vi "Broadcast Refnum Release.vi"(8 "error in":errorcluster) -> (0 "error out":errorcluster)   [LabVIEW 2020, in "SECS Scenarios.lvlib" / "Scenarios Class.lvclass"]
uses:
  Scenarios Class.lvclass
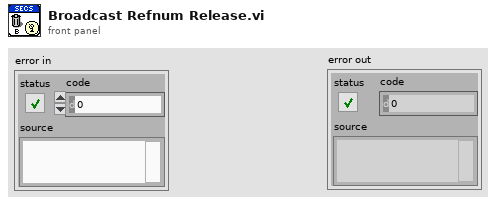
[diagram p1: front panel]
types:
  T1 = typedef "SECS Scenarios.lvlib/Scenarios Class.lvclass/Broadcast Refnum.ctl" = cluster{"13-EnableDisable Alarm":refnum<user-event>, "15-Process Program Request":refnum<user-event>, "16-Process Program Send":refnum<user-event>, "17-Deleting a Process Program by Host":refnum<user-event>, "18-Host Requests Equipment Process Program Directory":refnum<user-event>, "19-Equipment Process Program Uploading":refnum<user-event>, "20[1]-Process Program Downloading":refnum<user-event>, "20[2]-Process Program Downloading":refnum<user-event>, "22-Host Sends Information to Equipment":refnum<user-event>, "26-Host Requests to Enter OFF-Line":refnum<user-event>, "27-Host Requests to Enter On-Line":refnum<user-event>, "28[1]-Remote Control[PP-SELECT]":refnum<user-event>, "28[2]-Remote Control[START]":refnum<user-event>, "28[3]-Remote Control[STOP]":refnum<user-event>, "28[4]-Remote Control[LOCAL]":refnum<user-event>, "28[5]-Remote Control[REMOTE]":refnum<user-event>, "28[6]-Remote Control[RCMD]":refnum<user-event>, "30-Host Requests Equipment to Set Time":refnum<user-event>, "31-Host Requests Time Value from Equipment":refnum<user-event>, "32[1]-Trace Data Collection":refnum<user-event>, "32[2]-Trace Data Collection":refnum<user-event>}
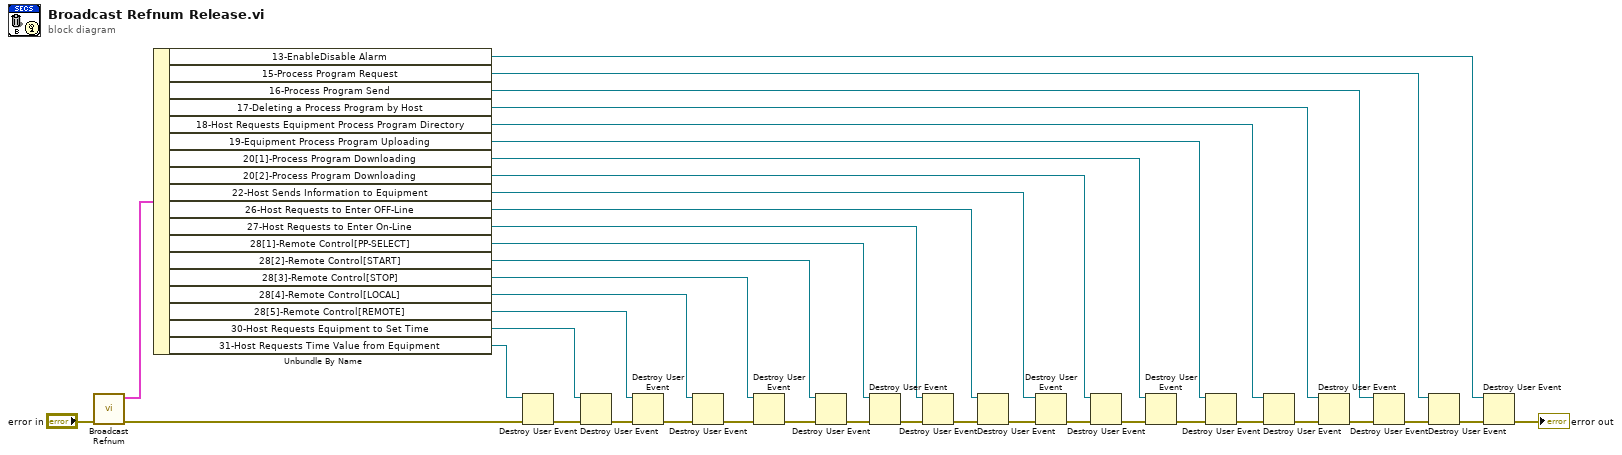
[diagram p0: block diagram]
diagram:
  n1 = call "Broadcast Refnum.vi"("error in"="error in") -> ("error out"=w1:errorcluster, "Broadcast Refnum"=w39:T1)  [unwired: 9 in]
  n2 = Unbundle By Name(w39) -> ("13-EnableDisable Alarm"=w35:refnum<user-event>, "15-Process Program Request"=w37:refnum<user-event>, "16-Process Program Send"=w29:refnum<user-event>, "17-Deleting a Process Program by Host"=w30:refnum<user-event>, "18-Host Requests Equipment Process Program Directory"=w31:refnum<user-event>, "19-Equipment Process Program Uploading"=w21:refnum<user-event>, "20[1]-Process Program Downloading"=w24:refnum<user-event>, "20[2]-Process Program Downloading"=w25:refnum<user-event>, "22-Host Sends Information to Equipment"=w26:refnum<user-event>, "26-Host Requests to Enter OFF-Line"=w18:refnum<user-event>, "27-Host Requests to Enter On-Line"=w16:refnum<user-event>, "28[1]-Remote Control[PP-SELECT]"=w14:refnum<user-event>, "28[2]-Remote Control[START]"=w12:refnum<user-event>, "28[3]-Remote Control[STOP]"=w10:refnum<user-event>, "28[4]-Remote Control[LOCAL]"=w8:refnum<user-event>, "28[5]-Remote Control[REMOTE]"=w6:refnum<user-event>, "30-Host Requests Equipment to Set Time"=w4:refnum<user-event>, "31-Host Requests Time Value from Equipment"=w2:refnum<user-event>)
  n3 = Destroy User Event(user event=w2, error in=w1) -> (error out=w3:errorcluster)
  n4 = Destroy User Event(user event=w4, error in=w3) -> (error out=w5:errorcluster)
  n5 = Destroy User Event(user event=w6, error in=w5) -> (error out=w7:errorcluster)
  n6 = Destroy User Event(user event=w8, error in=w7) -> (error out=w9:errorcluster)
  n7 = Destroy User Event(user event=w10, error in=w9) -> (error out=w11:errorcluster)
  n8 = Destroy User Event(user event=w12, error in=w11) -> (error out=w13:errorcluster)
  n9 = Destroy User Event(user event=w14, error in=w13) -> (error out=w15:errorcluster)
  n10 = Destroy User Event(user event=w16, error in=w15) -> (error out=w17:errorcluster)
  n11 = Destroy User Event(user event=w18, error in=w17) -> (error out=w19:errorcluster)
  n12 = Destroy User Event(user event=w26, error in=w19) -> (error out=w27:errorcluster)
  n13 = Destroy User Event(user event=w25, error in=w27) -> (error out=w28:errorcluster)
  n14 = Destroy User Event(user event=w24, error in=w28) -> (error out=w23:errorcluster)
  n15 = Destroy User Event(user event=w21, error in=w23) -> (error out=w22:errorcluster)
  n16 = Destroy User Event(user event=w31, error in=w22) -> (error out=w34:errorcluster)
  n17 = Destroy User Event(user event=w30, error in=w34) -> (error out=w33:errorcluster)
  n18 = Destroy User Event(user event=w29, error in=w33) -> (error out=w32:errorcluster)
  n19 = Destroy User Event(user event=w37, error in=w32) -> (error out=w36:errorcluster)
  n20 = Destroy User Event(user event=w35, error in=w36) -> (error out=→"error out":errorcluster)
